vi "Initialize Spectrometer.vi"(11 "Abstract Spectrometer in":refnum<class "Abstract Spectrometer.lvclass">) -> (0 "error out":errorcluster, 3 "Abstract Spectrometer out":refnum<class "Abstract Spectrometer.lvclass">)   [LabVIEW 2020, in "Spectrometer.lvlib"]
uses:
  Spectrometer.lvlib
  Spectrometer-LVClass/Abstract Spectrometer_class/Abstract Spectrometer.lvclass
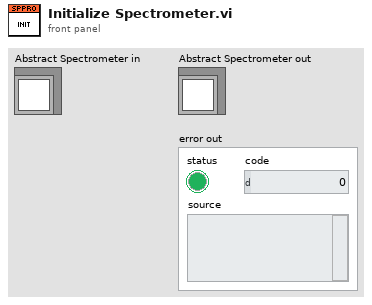
[diagram p1: front panel]
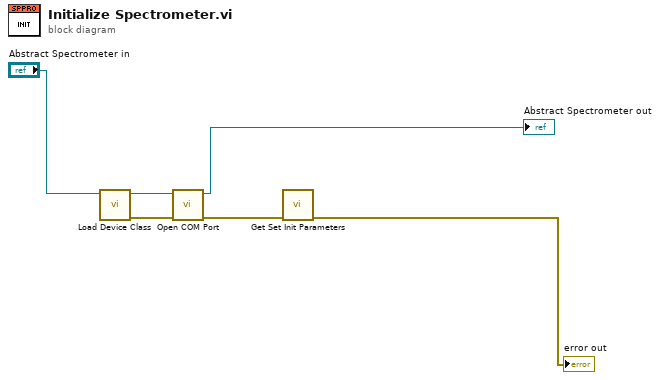
[diagram p0: block diagram]
diagram:
  n1 = call "Load Device Class.vi"("Abstract Spectrometer in"="Abstract Spectrometer in") -> ("error out"=w6:errorcluster, "Abstract Spectrometer out"=w3:refnum<class "Abstract Spectrometer.lvclass">)  [unwired: 9 in]
  n2 = call "Open COM Port.vi"("error in (no error)"=w6, "Abstract Spectrometer in"=w3) -> ("error out"=w4:errorcluster, "Abstract Spectrometer out"=→"Abstract Spectrometer out":refnum<class "Abstract Spectrometer.lvclass">)  [unwired: 8 in]
  n3 = call "Get Set Init Parameters.vi"("error in (no error)"=w4) -> ("error out"=→"error out":errorcluster)  [unwired: 10 in]
